vi "5.2 - Convert Theta Heading.vi"(1 "State Vector X Theta":dbl) -> (0 "Heading":dbl)   [LabVIEW 2010]
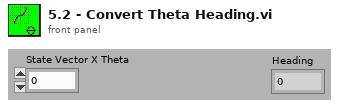
[diagram p1: front panel]
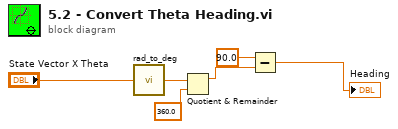
[diagram p0: block diagram]
diagram:
  n1 = call "rad_to_deg.vi"("Radians"="State Vector X Theta") -> ("Degrees"=w5:dbl)
  n2 = Quotient & Remainder(x=w5, y=360.0) -> (x-y*floor(x/y)=w3:dbl)  [unwired: 1 out]
  n3 = Subtract(x=90.0, y=w3) -> (x-y=→"Heading":dbl)
